vi "Read imported Profiles.vi"(7 "Target IP":string, 8 "error in":errorcluster, 9 "password":string, 10 "user name":string) -> (0 "error out":errorcluster, 2 "Existing Host Profiles":string[](array[string]), 3 "Existing Target Profiles":string[](array[string]))   [LabVIEW 2016, in "Scan Engine Custom Device.lvlib"]
uses:
  Scan Engine Custom Device.lvlib
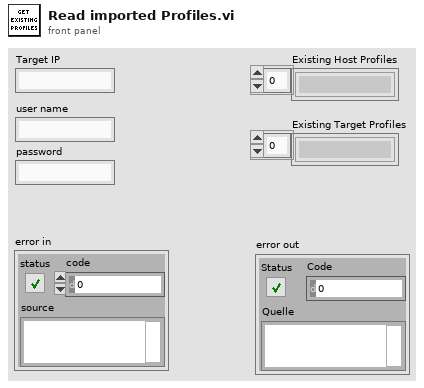
[diagram p1: front panel]
types:
  T1 = typedef "_fileTransferProtocol.ctl" = enum16{"Ftp", "WebDAV", "None"}
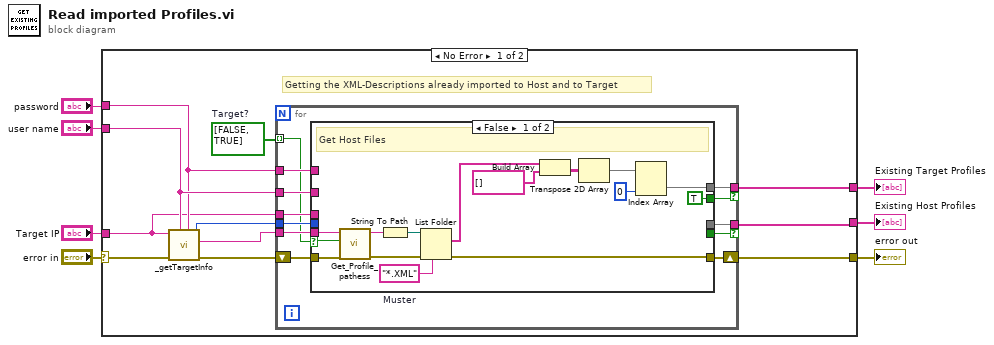
[diagram p0: block diagram]
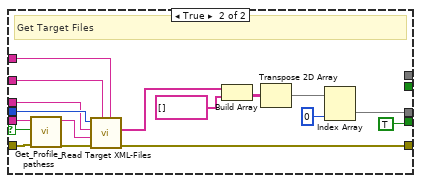
[diagram p2: hidden frame]
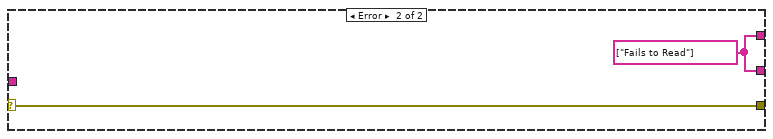
[diagram p3: hidden frame]
diagram:
  n1 = case shown="No Error" "error in" {
    selector: "error in" -> [w15 w64]
    tunnel: "Target IP" -> [w12 _]
    tunnel: "user name" -> [w14 _]
    tunnel: "password" -> [w13 _]
    tunnel: [w10 w64] -> w3
    tunnel: [w8 w63] -> w1
    tunnel: [w9 w63] -> w2
    frame No Error {
      w11 = bool[] [FALSE, TRUE]  # Target?
      # "Getting the XML-Descriptions already imported to Host and to Target"
      n2 = call <resource>:"_getTargetInfo.vi"("password"=w13, "user name"=w14, "error in"=w15, "Target IP"=w12) -> ("error out"=w18:errorcluster, "Target OS"=w16:string, "protocol"=w17:T1)  [unwired: 4 in, 1 out]
      n3 = for {
        tunnel: w17 -> [w29]
        tunnel: w16 -> [w27]
        tunnel: w14 -> [w26]
        tunnel: w13 -> [w25]
        tunnel: w12 -> [w24]
        shift-right: [w28] -> w10
        shift-left: w18 -> [w30]
        tunnel: w11 -> [w23] mode=indexing
        tunnel: [w22] -> w8 if=w21
        tunnel: [w20] -> w9 if=w19
        n4 = case shown="False" w23 {
          selector: w23 -> [w44 w56]
          tunnel: w30 -> [w45 w62]
          tunnel: w29 -> [_ w61]
          tunnel: [w38 w59] -> w28
          tunnel: w27 -> [w43 w58]
          tunnel: w26 -> [_ w55]
          tunnel: w25 -> [_ w54]
          tunnel: w24 -> [_ w53]
          tunnel: [_ w47] -> w22
          tunnel: [_ TRUE] -> w21
          tunnel: [w32 _] -> w20
          tunnel: [TRUE _] -> w19
          frame False {
            w42 = "*.XML"  # Muster
            # "Get Host Files"
            n5 = call "Get_Profile_pathess.vi"("error in (no error)"=w45, "Target?"=w44, "OSArch"=w43) -> ("error out"=w39:errorcluster, "profileDestPath"=w40:string)  [unwired: 7 in]
            n6 = String To Path(string=w40) -> (path=w41:path)
            n7 = List Folder(path=w41, pattern=w42, error in=w39) -> (filenames=w35:string[], error out=w38:errorcluster)  [unwired: 1 in, 2 out]
            n8 = Build Array(w35, string[] [] ("Element")) -> (w37:string[][])
            n9 = Transpose 2D Array(2D array=w37) -> (transposed array=w33:string[][])
            n10 = Index Array(array=w33, index (col)=0) -> (element=w32:string[])  [unwired: 1 in]
          }
          frame True {
            # "Get Target Files"
            n11 = call "Get_Profile_pathess.vi"("error in (no error)"=w62, "Target?"=w56, "OSArch"=w58) -> ("error out"=w60:errorcluster, "profileDestPath"=w57:string)  [unwired: 7 in]
            n12 = call "Read Target XML-Files.vi"("password"=w54, "user name"=w55, "error in (no error)"=w60, "ddDestPath in"=w57, "Target IP"=w53, "protocol"=w61) -> ("error out"=w59:errorcluster, "Fies"=w50:string[])  [unwired: 3 in, 1 out]
            n13 = Build Array(w50, string[] [] ("Element")) -> (w52:string[][])
            n14 = Transpose 2D Array(2D array=w52) -> (transposed array=w48:string[][])
            n15 = Index Array(array=w48, index (col)=0) -> (element=w47:string[])  [unwired: 1 in]
          }
        }
      }
    }
    frame Error {
      w63 = string[] ["Fails to Read"]
    }
  }
  "error out" <- w3
  "Existing Host Profiles" <- w1
  "Existing Target Profiles" <- w2
